vi "Go to field (immediately).vi"(8 "error in":errorcluster, 10 "Desired field (T)":dbl[unit], 11 "varian in":refnum<class "Varian Magnet.lvclass">) -> (0 "error out":errorcluster, 3 "varian out":refnum<class "Varian Magnet.lvclass">)   [LabVIEW 2009, in "Varian Magnet.lvclass"]
doc: "Sets the control voltage based on the Long-Term Field Calibration in Varian Constants.vi Global."
uses:
  Varian Magnet.lvclass
  Varian Magnet.lvclass/Varian Magnet.ctl
  Varian Constants.vi
  <vilib>/gmath/NI_Gmath.lvlib
  Varian/Varian.lvlib
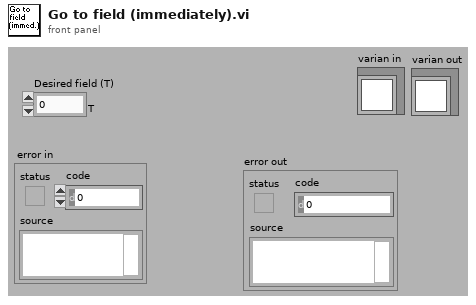
[diagram p1: front panel]
types:
  T1 = typedef "NI_Gmath.lvlib/in_piecewise interp poly control.ctl" = cluster{"x locations":dbl[], "coefficients":dbl[][]}
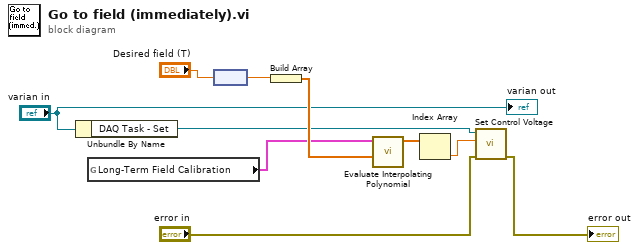
[diagram p0: block diagram]
diagram:
  n1 = Unbundle By Name("varian in") -> ("DAQ Task - Set"=w5:refnum<k21>)
  n2 = global read "Varian Constants.vi" "Long-Term Field Calibration"() -> (w7:T1)
  n3 = node("Desired field (T)") -> (w9:dbl)
  n4 = Build Array(w9) -> (w8:dbl[])
  n5 = call <vilib>:"Evaluate Interpolating Polynomial.vi"("xi"=w8, "piecewise polynomial"=w7) -> ("yi"=w6:dbl[])  [unwired: 8 in, 1 out]
  n6 = Index Array(array=w6) -> (element=w4:dbl)  [unwired: 1 in]
  n7 = call "Set Control Voltage.vi"("error in"="error in", "Control Voltage"=w4, "task in"=w5) -> ("error out"=→"error out":errorcluster)  [unwired: 7 in, 1 out]
  "varian out" <- "varian in"
